vi "DAISY_Polarity_sign_array.vi"(8 "error in (no error)":errorcluster[](array[cluster]), 11 "BoardHandles":T1(array[cluster])) -> (0 "Errors Out":errorcluster[](array[cluster]), 1 "Polarity signs":i32[](array[numeric]), 3 "Board Handles Out":T1(array[cluster]))   [LabVIEW 2018]
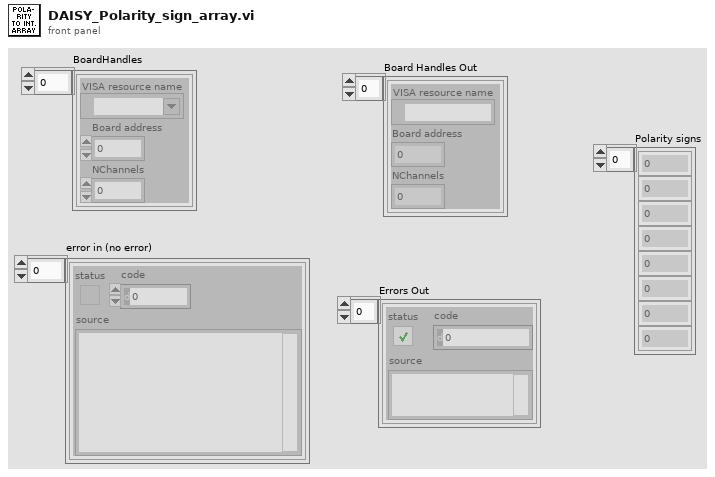
[diagram p1: front panel]
types:
  T1 = cluster{"VISA resource name":refnum<visa-resource-name>, "Board address":u8, "NChannels":u8}[]
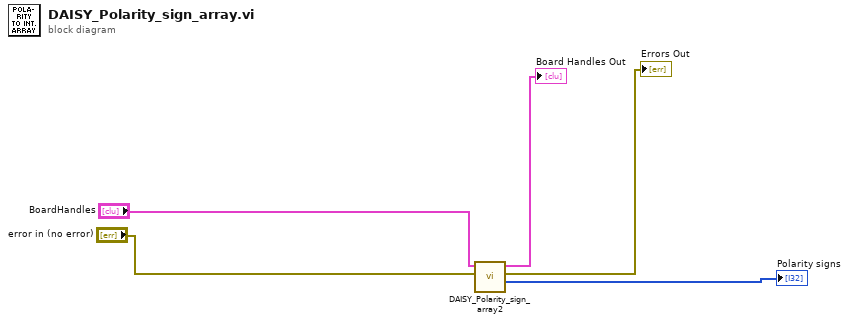
[diagram p0: block diagram]
diagram:
  n1 = call "DAISY_Polarity_sign_array2.vi"("error in (no error)"="error in (no error)", "BoardHandle"="BoardHandles") -> ("Array"=→"Polarity signs":i32[], "Array 2"=→"Errors Out":errorcluster[], "Array 3"=→"Board Handles Out":T1)  [unwired: 7 in]
